vi "Tester.vi"() -> ()   [LabVIEW 2026, in "GH2.lvclass"]
uses:
  GH2.lvclass
panel:
  in  "send":bool
  out "error out":errorcluster
  out "Response":string
  in  "Command Input":string
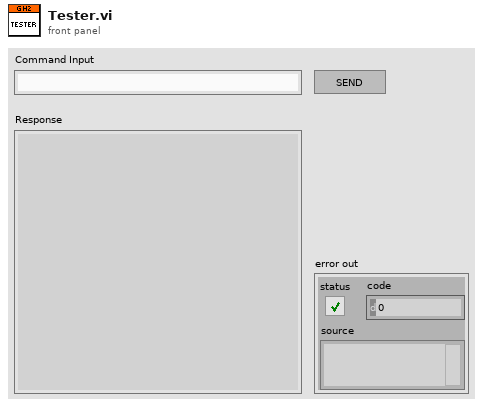
[diagram p1: front panel]
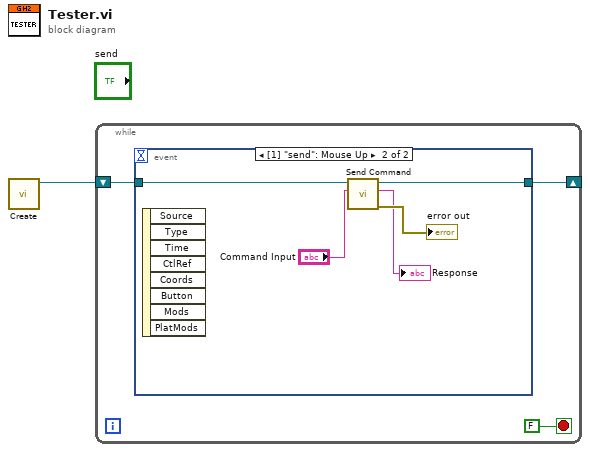
[diagram p0: block diagram]
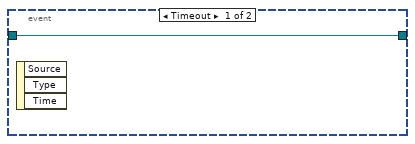
[diagram p2: hidden frame]
diagram:
  n1 = call "Create.vi"() -> ("GH2 out"=w1:refnum<class "GH2.lvclass">)  [unwired: 10 in, 1 out]
  n2 = while {
    shift-right: [w3] -> _
    shift-left: w1 -> [w4]
    stop <- FALSE stop-if-true
    n3 = event shown="[1] \"send\": Mouse Up" {
      selector: _ -> [_ _]
      dyn-events: _ -> [_ _]
      timeout: _ -> [_ _]
      tunnel: w4 -> [w5 w7]
      tunnel: [w5 w6] -> w3
      event Timeout {
        n4 = event-data() -> ()  [unwired: 1 in, 3 out]
      }
      event "send": Mouse Up {
        n5 = event-data() -> ()  [unwired: 1 in, 8 out]
        n6 = call "Send Command.vi"("command"="Command Input", "GH2 in"=w7) -> ("error out"=→"error out":errorcluster, "response"=→"Response":string, "GH2 out"=w6:refnum<class "GH2.lvclass">)  [unwired: 7 in]
      }
    }
  }
